vi "Init.vi"(5 "EventLogger":refnum<class "EventLoggingService.lvclass">, 8 "error in (no error)":errorcluster, 9 "Node":string, 10 "Cluster":string, 11 "System":string) -> (0 "error out":errorcluster, 3 "ChannelService out":refnum<class "ChannelService.lvclass">)   [LabVIEW 2020, in "Vecto.lvlib" / "ChannelService.lvclass"]
uses:
  ChannelService.lvclass
  EventLoggingService/EventLoggingService.lvclass
  Event Level.ctl
  ChannelService.lvclass/ChannelService.ctl
  EventLoggingService/EventLoggingService.lvclass/EventLoggingService.ctl
  <vilib>/Utility/error.llb/Error Cluster From Error Code.vi
  EventLogHandler/EventLogHandler.lvclass
  Vecto.lvlib
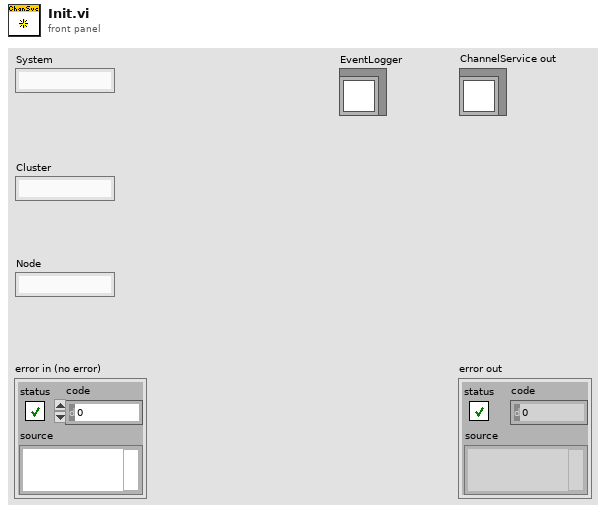
[diagram p1: front panel]
types:
  T1 = typedef "Vecto.lvlib/Event Level.ctl" = enum16{"Debug", "Info", "Warning", "Error"}
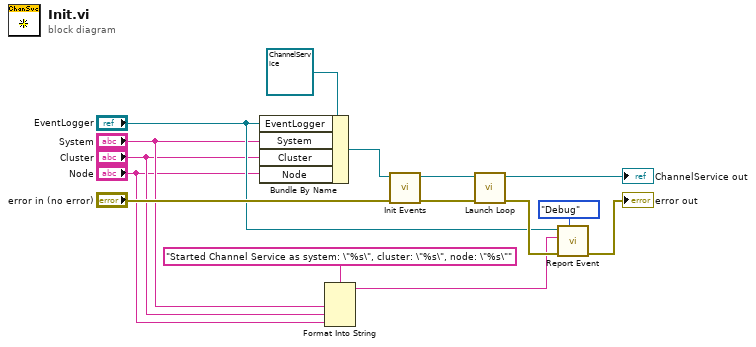
[diagram p0: block diagram]
diagram:
  n1 = Bundle By Name(cluster=refnum<class "ChannelService.lvclass"> refnum ("ChannelService in"), "EventLogger"="EventLogger", "System"="System", "Cluster"="Cluster", "Node"="Node") -> (w11:refnum<class "ChannelService.lvclass">)
  n2 = Format Into String(format string="Started Channel Service as system: \"%s\", cluster: \"%s\", node: \"%s\"", "System", "Cluster", "Node") -> (resulting string=w2:string)  [unwired: 2 in, 1 out]
  n3 = call "Init Events.vi"("error in (no error)"="error in (no error)", "ChannelService in"=w11) -> ("error out"=w12:errorcluster, "ChannelService out"=w10:refnum<class "ChannelService.lvclass">)  [unwired: 8 in]
  n4 = call "Launch Loop.vi"("error in (no error)"=w12, "ChannelService in"=w10) -> ("error out"=w15:errorcluster, "ChannelService out"=→"ChannelService out":refnum<class "ChannelService.lvclass">)  [unwired: 8 in]
  n5 = call "Report Event.vi"("Event Level (Info)"=Event_Level."Debug", "error in (no error)"=w15, "Message"=w2, "EventLoggingService in"="EventLogger") -> ("error out"=→"error out":errorcluster)  [unwired: 6 in, 1 out]
